vi "Sort spreadsheet with date format fix.vi"(7 "Date field?":bool, 8 "error in (no error)":errorcluster, 9 "Descending (F)":bool, 10 "Priority Columns (0)":i32[](array[numeric])=[0], 11 "Unsorted Spreadsheet":string[][](array[string])) -> (0 "error out":errorcluster, 3 "Sorted Spreadsheet":string[][](array[string]))   [LabVIEW 2013]
panel:
  out "Spreadsheet date fixed":string[][](array[string])
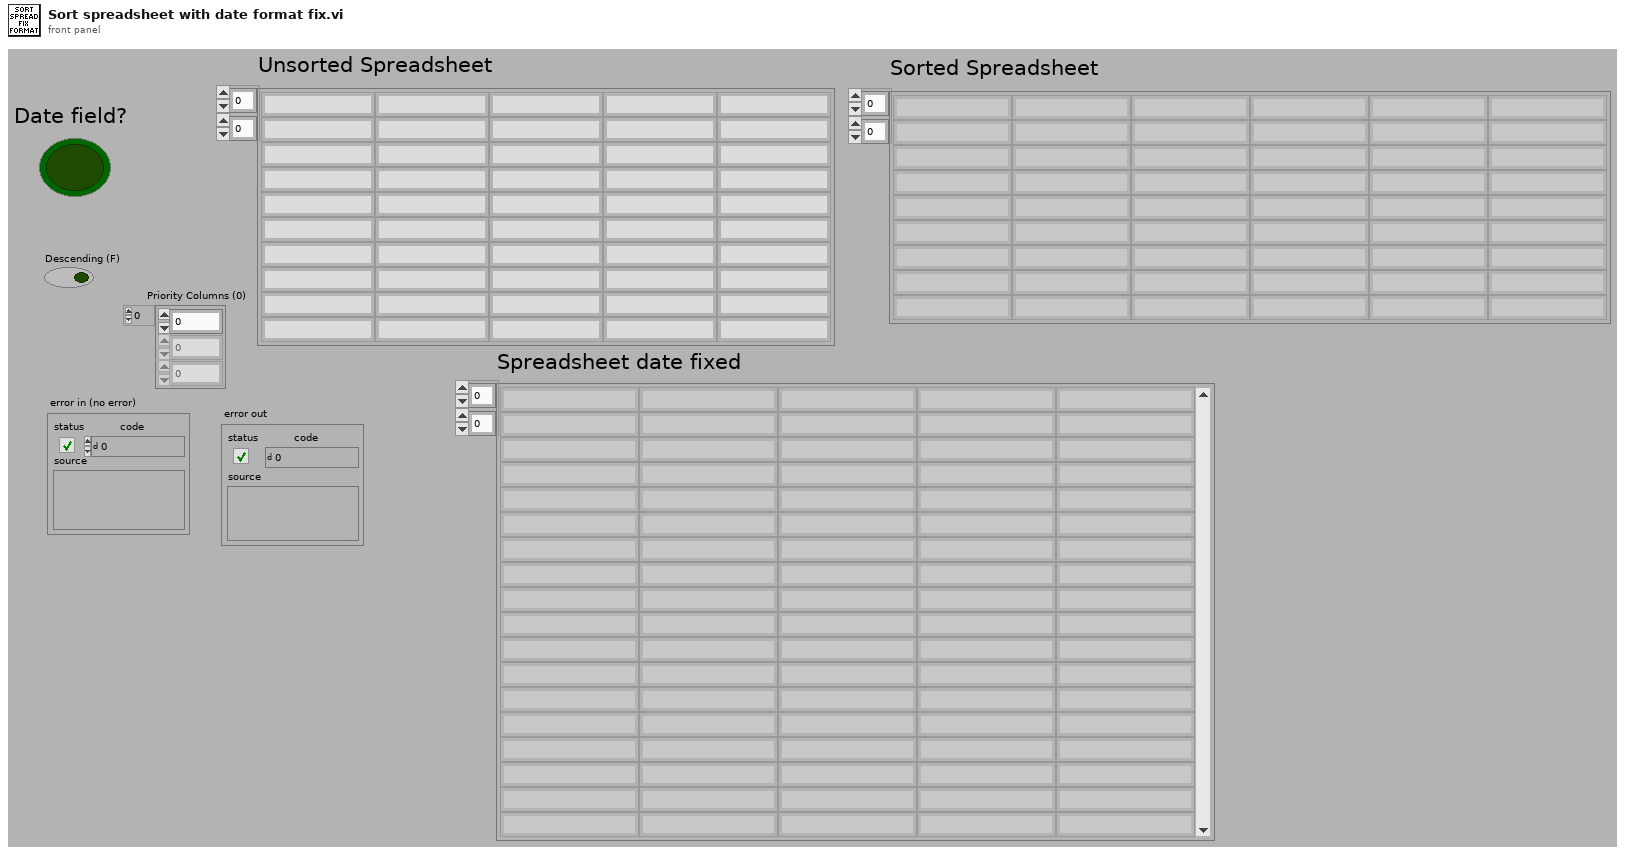
[diagram p1: front panel]
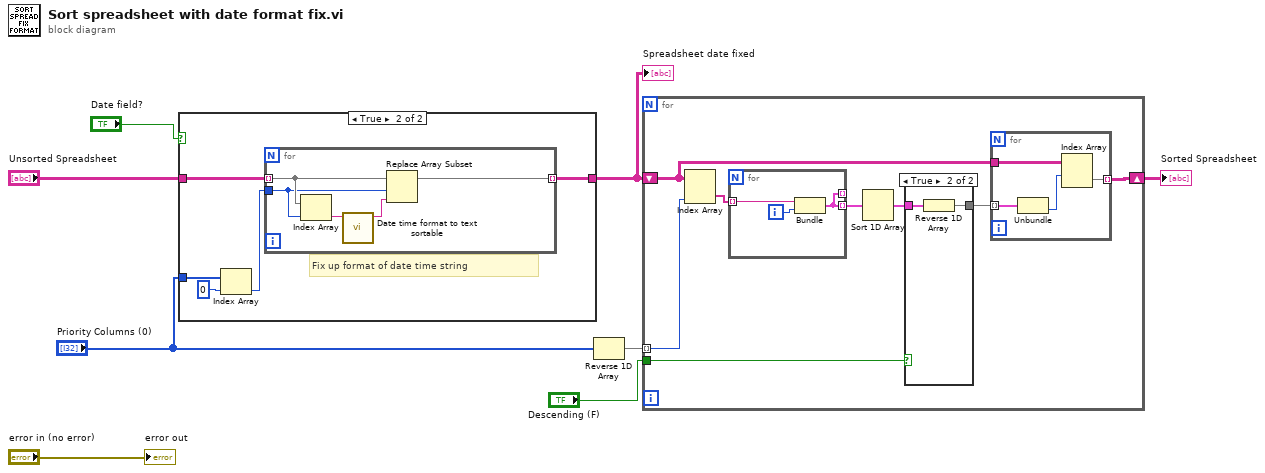
[diagram p0: block diagram]
diagram:
  n1 = case shown="True" "Date field?" {
    tunnel: "Priority Columns (0)" -> [_ w14]
    tunnel: "Unsorted Spreadsheet" -> [w9 w11]
    tunnel: [w9 w10] -> w2
    frame False {
    }
    frame True {
      # "Fix up format of date time string"
      n2 = Index Array(array=w14, index=0) -> (element=w12:i32)
      n3 = for {
        tunnel: w12 -> [w17]
        tunnel: w11 -> [w18] mode=indexing
        tunnel: [w15] -> w10 mode=indexing
        n4 = Index Array(array=w18, index=w17) -> (element=w19:string)
        n5 = call "Date time format to text sortable.vi"("Date time string"=w19) -> ("New date time string"=w16:string)  [unwired: 9 in, 1 out]
        n6 = Replace Array Subset(array=w18, new element=w16, index=w17) -> (w15:string[])
      }
    }
  }
  "Spreadsheet date fixed" <- w2
  n7 = Reverse 1D Array(array="Priority Columns (0)") -> (reversed array=w8:i32[])
  n8 = for {
    shift-right: [w22] -> w1
    shift-left: w2 -> [w24]
    tunnel: w8 -> [w21] mode=indexing
    tunnel: "Descending (F)" -> [w23]
    n9 = Index Array(array=w24, index (col)=w21) -> (element=w25:string[])  [unwired: 1 in]
    n10 = for {
      tunnel: w25 -> [w36] mode=indexing
      tunnel: [w35] -> _ mode=indexing
      tunnel: [w35] -> w20 mode=indexing
      i -> [w37]
      n11 = Bundle("String"=w36, w37) -> (w35:cluster{"String":string, i32})  [unwired: 1 out]
    }
    n12 = Sort 1D Array(array=w20) -> (sorted array=w27:cluster{"String":string, i32}[])
    n13 = case shown="True" w23 {
      tunnel: [w28 w29] -> w26
      tunnel: w27 -> [w28 w30]
      frame False {
      }
      frame True {
        n14 = Reverse 1D Array(array=w30) -> (reversed array=w29:cluster{"String":string, i32}[])
      }
    }
    n15 = for {
      tunnel: w26 -> [w32] mode=indexing
      tunnel: w24 -> [w34]
      tunnel: [w33] -> w22 mode=indexing
      n16 = Unbundle(w32) -> (w31:i32)  [unwired: 1 out]
      n17 = Index Array(array=w34, index (row)=w31) -> (element=w33:string[])  [unwired: 1 in]
    }
  }
  "Sorted Spreadsheet" <- w1
  "error out" <- "error in (no error)"
